vi "Get Attribute Name from Tag.vi"(11 "Tag":string) -> (1 "Linked List":bool, 2 "Linked List ID":string, 3 "Attribute Name":string)   [LabVIEW 2020, in "Linked Lists.lvlib" / "Linked List.lvclass"]
uses:
  <vilib>/gpm_packages/@cs/linked-list/Source/Linked List/Linked List/Linked List.lvclass
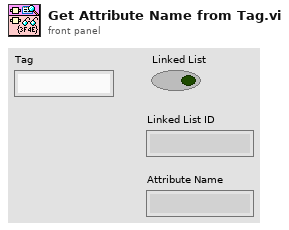
[diagram p1: front panel]
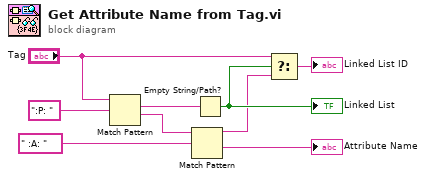
[diagram p0: block diagram]
diagram:
  n1 = Match Pattern(string="Tag", regular expression=":P: " ("string")) -> (match substring=w6:string, after substring=w7:string)  [unwired: 1 in, 2 out]
  n2 = Match Pattern(string=w7, regular expression=" :A: " ("string")) -> (before substring=w1:string, after substring=→"Attribute Name":string)  [unwired: 1 in, 2 out]
  n3 = Empty String/Path?(string/path=w6) -> (empty?=w4:bool)
  "Linked List" <- w4
  n4 = Select(t="Tag", s=w4, f=w1) -> (s? t:f=→"Linked List ID":string)
